vi "Test Refresh Active Rectangle is First.vi"(8 "error in (no error)":errorcluster) -> (0 "error out":errorcluster)   [LabVIEW 2019]
uses:
  <vilib>/addons/_JKI Toolkits/Caraya/classes/Assert/Assert.lvclass
  Setting Database/Setting Database.lvclass
  <vilib>/JKI/JKI SMO/SMO/SMO.lvclass
  C:/Program Files (x86)/National Instruments/LabVIEW 2019/vi.lib/JKI/JKI SMO/SMO/SMO.lvclass
  <vilib>/addons/_JKI Toolkits/Caraya/classes/Assert/Assert Equal Value_Variant.vi
  Rectangle Settings/Rectangle Settings.lvclass
  C:/Users/Albro/Documents/GitHub/AFM-Lithography/lvsrc/Classes/Settings/ObjectSettings/ObjectSettings.lvclass
  <vilib>/addons/_JKI Toolkits/Caraya/classes/Test/Test.lvclass
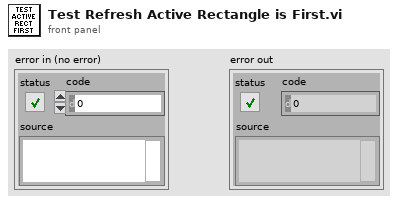
[diagram p1: front panel]
types:
  T1 = typedef "Setting Database.lvclass/PublicEvents--Cluster.ctl" = cluster{"NewActivePath":refnum<user-event>, "PathsUpdated":refnum<user-event>, "RectanglesUpdated":refnum<user-event>, "NewActiveRectangle":refnum<user-event>, "NewActiveFunnel":refnum<user-event>, "FunnelsUpdated":refnum<user-event>, "NewActiveDot":refnum<user-event>, "DotsUpdated":refnum<user-event>}
  T2 = typedef "Setting Database.lvclass/PrivateEvents--Setting Database.Refresh.ctl" = cluster{"Paths":string[], "Rectangles":string[], "Funnels":string[], "Dots":string[]}
  T3 = typedef "Setting Database.lvclass/PublicEvents--Setting Database.NewActiveRectangle.ctl" = refnum<class "Rectangle Settings.lvclass">
  T4 = typedef "Setting Database.lvclass/PublicEvents--Setting Database.RectanglesUpdated.ctl" = refnum<class "Rectangle Settings.lvclass">[]
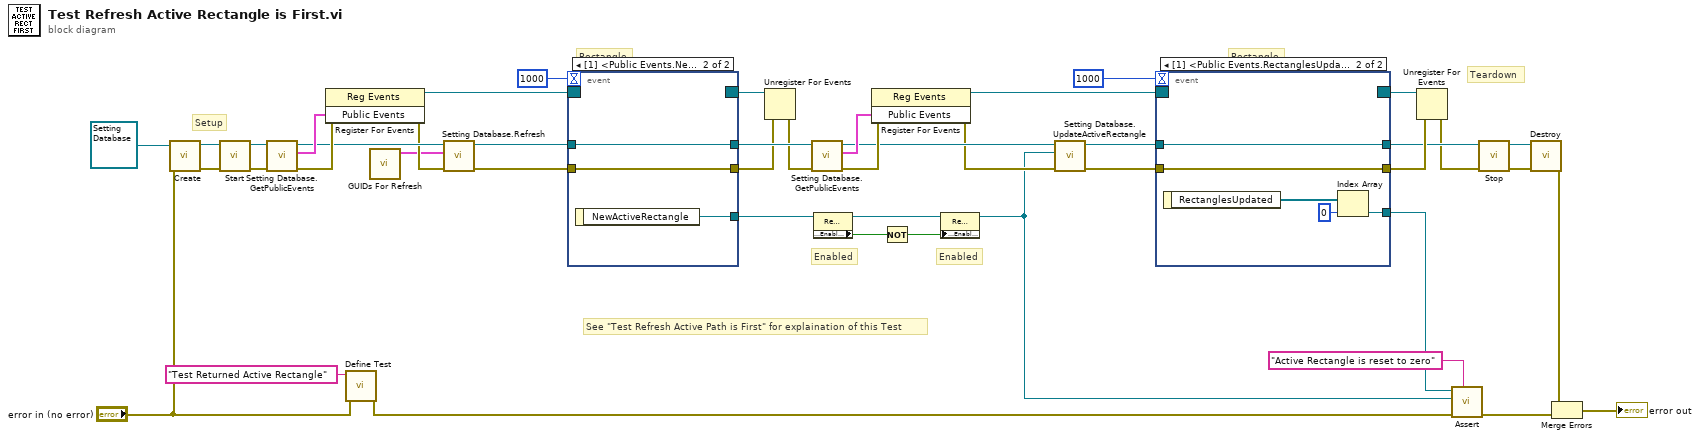
[diagram p0: block diagram]
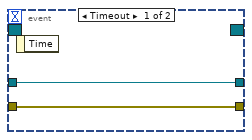
[diagram p2: hidden frame]
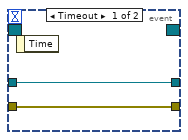
[diagram p3: hidden frame]
diagram:
  # "See \"Test Refresh Active Path is First\" for explaination of this Test"
  # "Enabled"
  # "Enabled"
  # "Rectangle"
  # "Rectangle"
  # "Teardown"
  # "Setup"
  n1 = call <vilib>:"Create.vi"("error in (no error)"="error in (no error)", "SMO"=refnum<class "Setting Database.lvclass"> refnum ("Setting Database.lvclass")) -> ("error out"=w43:errorcluster, "SMO out"=w37:refnum<class "Setting Database.lvclass">)  [unwired: 7 in, 1 out]
  n2 = call <vilib>:"Start.vi"("error in (no error)"=w43, "SMO"=w37) -> ("error out"=w42:errorcluster, "SMO out"=w36:refnum<class "Setting Database.lvclass">)  [unwired: 8 in]
  n3 = call "Setting Database.GetPublicEvents.vi"("error in (no error)"=w42, "Setting Database"=w36) -> ("error out"=w40:errorcluster, "Public Events"=w32:T1, "Setting Database out"=w30:refnum<class "Setting Database.lvclass">)  [unwired: 7 in]
  n4 = register-events(error in=w40, w32) -> (reference out=w31:refnum<event-registration>, error out=w28:errorcluster)  [unwired: 1 in]
  n5 = call <vilib>:"Define Test.vi"("error in (no error)"="error in (no error)", "Label (VI Title)"="Test Returned Active Rectangle") -> ("error out"=w3:errorcluster)  [unwired: 8 in, 1 out]
  n6 = call "GUIDs For Refresh.vi"() -> ("Initialize"=w1:T2)  [unwired: 11 in]
  n7 = call "Setting Database.Refresh.vi"("error in (no error)"=w28, "Initialize"=w1, "Setting Database"=w30) -> ("error out"=w27:errorcluster, "Setting Database out"=w29:refnum<class "Setting Database.lvclass">)  [unwired: 7 in]
  n8 = event shown="[1] <Public Events.NewActiveRectangle>: User Event" {
    selector: w31 -> [_ _]
    dyn-events: [_ _] -> w34
    timeout: 1000 -> [_ _]
    tunnel: [w47 w50] -> w25
    tunnel: w27 -> [w47 w50]
    tunnel: w29 -> [w46 w49]
    tunnel: [w46 w49] -> w26
    tunnel: [_ w48] -> w15
    event Timeout {
      n9 = event-data() -> ()  [unwired: 1 in, 1 out]
    }
    event User Event {
      n10 = event-data() -> ("NewActiveRectangle"=w48:T3)  [unwired: 1 in]
    }
  }
  n11 = Unregister For Events(event registration refnum=w34, error in=w25) -> (error out=w24:errorcluster)
  n12 = call "Setting Database.GetPublicEvents.vi"("error in (no error)"=w24, "Setting Database"=w26) -> ("error out"=w22:errorcluster, "Public Events"=w23:T1, "Setting Database out"=w9:refnum<class "Setting Database.lvclass">)  [unwired: 7 in]
  n13 = property class="Rectangle Settings.lvclass"(reference=w15) -> (reference out=w14:T3, "Accessors:Enabled"=w13:bool)  [unwired: 1 in, 1 out]
  n14 = register-events(error in=w22, w23) -> (reference out=w18:refnum<event-registration>, error out=w7:errorcluster)  [unwired: 1 in]
  n15 = Not(x=w13) -> (.not. x?=w12:bool)
  n16 = property class="Rectangle Settings.lvclass"(reference=w14, "Accessors:Enabled"=w12) -> (reference out=w5:T3)  [unwired: 1 in, 1 out]
  n17 = call "Setting Database.UpdateActiveRectangle.vi"("error in (no error)"=w7, "UpdateActiveRectangle"=w5, "Setting Database"=w9) -> ("error out"=w6:errorcluster, "Setting Database"=w8:refnum<class "Setting Database.lvclass">)  [unwired: 7 in]
  n18 = event shown="[1] <Public Events.RectanglesUpdated>: User Event" {
    selector: w18 -> [_ _]
    dyn-events: [_ _] -> w19
    timeout: 1000 -> [_ _]
    tunnel: [w52 w57] -> w21
    tunnel: w6 -> [w52 w57]
    tunnel: w8 -> [w51 w56]
    tunnel: [w51 w56] -> w17
    tunnel: [_ w54] -> w11
    event Timeout {
      n19 = event-data() -> ()  [unwired: 1 in, 1 out]
    }
    event User Event {
      n20 = event-data() -> ("RectanglesUpdated"=w55:T4)  [unwired: 1 in]
      n21 = Index Array(array=w55, index=0) -> (element=w54:refnum<class "Rectangle Settings.lvclass">)
    }
  }
  n22 = Unregister For Events(event registration refnum=w19, error in=w21) -> (error out=w16:errorcluster)
  n23 = call-poly <vilib>:"Assert.vi"("Label"="Active Rectangle is reset to zero", "error in (no error)"=w3, "Actual"=w5, "Expected"=w11) -> ("error out"=w45:errorcluster)  [unwired: 6 in, 1 out]
  n24 = call <vilib>:"Stop.vi"("error in (no error)"=w16, "SMO"=w17) -> ("error out"=w41:errorcluster, "SMO out"=w35:refnum<class "Setting Database.lvclass">)  [unwired: 8 in]
  n25 = call <vilib>:"Destroy.vi"("error in (no error)"=w41, "SMO"=w35) -> ("error out"=w39:errorcluster)  [unwired: 9 in]
  n26 = Merge Errors(w39, w45) -> (→"error out":errorcluster)
